vi "sub_hw-set.vi"(7 "cmd":T1=enum."AO 0v", 8 "error in":errorcluster, 10 "DUT Ch":i32, 11 "onoff":bool) -> (0 "error out":errorcluster)   [LabVIEW 2019]
uses:
  hw-control.ctl
  cmd_timer.ctl
  _ctrl/rw.ctl
  Devices/NI Board/cDAQ-9269 AO/type_signal.ctl
  Durability/common/UI.ctl
  Devices/NI Board/cDAQ-9476 DO/cnt_Relay.ctl
  Devices/NI Board/cDAQ-9476 DO/cnt_do.ctl
  Durability/common/cmd_timecheck.ctl
  _ctrl/BP4610_config.ctl
  _ctrl/BP4610_cmd.ctl
  _ctrl/DSP_action.ctl
  _ctrl/create-rw-close.ctl
  _ctrl/start.ctl
  _ctrl/fgv_DL950.ctl
  cmd_offtimecheck.ctl
  _ctrl/system-status.ctl
  _ctrl/init-r-stop.ctl
  4ec001e4-0f3b-4ebf-849a-f4f83a7bab7c.vi
  e6889d7c-de11-414d-a0e0-4227c0c1917b.vi
  0bae8188-c8c3-4ffc-ad07-b2da4a811416.vi
  23ae199e-3a96-4767-bc63-b89c967d0f14.vi
  470acc9e-1f4f-4ee6-a90f-225dc51f797d.vi
  0dce9dd1-3bd9-4495-8249-675a9cbc74d0.vi
  06f06628-476d-4804-93c1-d30ef29838a9.vi
  9f7e44c7-c157-4d85-83aa-43634e971710.vi
  Glob_Ref.vi
  Durability/common/Global 1.vi
  34f4878d-8da2-4261-96f6-505d6876a221.vi
  e9941be1-5017-49c9-9991-91539d334db2.vi
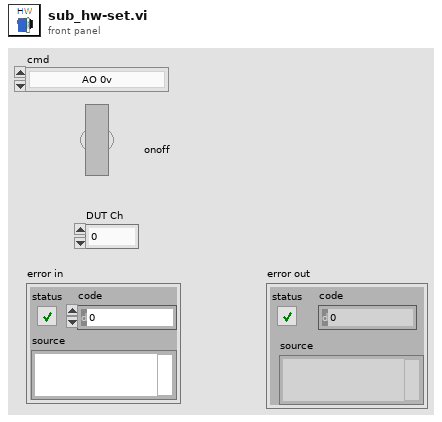
[diagram p1: front panel]
types:
  T1 = typedef "hw-control.ctl" = enum16{"DL950 ready", "DL950 clear", "DL950 trigger", "DL950 read", "DL950 read seq", "DL950 Tsingle query", "AO 12v", "AO wave", "AO 0v", "relay all-off", "Discharge check", "Discharge", "Relay1", "Relay2", "Relay3", "Relay4", "Relay5", "Relay6", "BP4610 onoff", "BP4610 set", "DSP1500 set", "DSP1500 onoff"}
  T2 = typedef "rw.ctl" = enum16{"read", "write"}
  T3 = typedef "cmd_timer.ctl" = enum16{"init", "init_update", "run", "default", "update"}
  T4 = typedef "cap_config.ctl" = cluster{"Test Mode":enum32{"6.3.2 저온 작동/방치 시험", "6.3.3 고온 작동/방치 시험", "6.3.4 온도 싸이클 시험", "6.3.6 온습도 싸이클 시험", "6.3.8 결로 시험", "6.3.9 빙결 시험"}, "ON time[ms]":dbl, "OFF time[ms]":dbl, "1. 작동시간[분]":dbl, "2. 미작동시간[분]":dbl, "3. 작동시간[분]":dbl, "level[V]":dbl, "duty":dbl, "Freq":dbl, "Voltage+[V]":dbl, "Voltage-[V]":dbl, "Current+[A]":dbl, "Current-[A]":dbl, "출력전압[V]":dbl, "출력전류[A]":dbl, "OVP Level":dbl, "OCP Level":dbl, "Time Div":u16, "Record Len":i32, "방전 기준[V]":dbl, "Repeate (Each Ch)":u32, "Cycle[N]":u32, "ON/OFF 회 수[N]":dbl, "TrigPos[%]":dbl, "시험시간[분]":dbl}
  T5 = typedef "Testing-info.ctl" = cluster{"전체채널수":u8, "현재채널번호":u8, "Irms":dbl, "입력전압":dbl, "입력전류":dbl, "출력전압":dbl, "출력전류":dbl, "온도":dbl, "제어단 단선":bool, "제어단 단락":bool, "제어단 특성변화":bool, "출력단 단선":bool, "출력단 단락":bool, "출력단 특성변화":bool, "출력단 전압":bool, "카운트 일치":bool, "Irms 판정":bool, "온도":bool, "테스트 회수":u32, "TestType":T6, "현재회수":u32, "Ch selection":cluster{"1ch":bool, "2ch":bool, "3ch":bool, "4ch":bool, "5ch":bool, "6ch":bool}, "반복":u32, "Path":path, "파일생성주기":u32, "start time":dbl, "stop time":dbl, "현재반복회수":u32, "NG":cluster{"입출력 카운트":bool, "출력전류RMS":bool}}
  T6 = typedef "sequence_single.ctl" = enum16{"Register", "RC", "B1", "B2", "B3", "Oper_LV", "Oper_HV", "ContR_LV"}
  T7 = typedef "type_signal.ctl" = enum16{"wave", "level"}
  T8 = typedef "UI.ctl" = enum16{"Alarm yellow", "DL950 graph show", "DL950 graph clear", "AO value", "AO blink onoff", "Discharge relay", "Input Power", "Outpower", "Relay in1", "Relay in2", "Relay in3", "Relay in4", "Relay in5", "Relay in6", "Relay out1", "Relay out2", "Relay out3", "Relay out4", "Relay out5", "Relay out6", "Relay all off"}
  T9 = typedef "cmd_timecheck.ctl" = enum16{"Group start", "Group end", "Grout dt", "Ch start", "Ch end", "Ch dt", "init", "NF start", "NF stop", "idrc start", "idrc stop", "scope start", "scope stop", "ao start", "ao stop", "relay start", "relay stop", "NF read start", "NF read stop", "NF set start", "NF set stop", "idrc level start", "idrc level stop", "scope trig start", "scope trig stop", "relay dischar star", "relay dischar stop", "data process start", "data process stop", "ch-relay on start", "ch-relay on stop", "hw set start", "hw set stop", "pwr-in on start", "pwr-in on stop", "pwr-out on start", "pwr-out on stop", "ao on start", "ao on stop", "ao 0v start", "ao 0v stop", "pwr-in off start", "pwr-in off stop", "relay-all off start", "relay-all off stop", "pwr-out off start", "pwr-out off stop", "discharge start", "discharge stop", "950 read start", "950 read stop"}
  T10 = typedef "cnt_do.ctl" = enum16{"open", "initial", "update", "run", "close"}
  T11 = typedef "cnt_Relay.ctl" = enum32{"R_Load", "R_out1", "R_out2", "R_out3", "R_out4", "R_out5", "R_out6", "R8", "R9", "R10", "R11", "R12", "R13", "R14", "R15", "R16", "R_in1", "R_in2", "R_in3", "R_in4", "R_in5", "R_in6", "R23", "R24", "R25", "R26", "R27", "R_red", "R_yellow", "R_green", "R_buz", "R_purple"}
  T12 = typedef "BP4610_cmd.ctl" = enum16{"open", "read", "set", "set_seq", "limit", "limit_seq", "output on", "output off", "close"}
  T13 = typedef "BP4610_config.ctl" = cluster{"VISA":refnum<visa-resource-name>, "Limit-BP":cluster{"Set":enum16{"Current", "Voltage"}, "Voltage+[V]":dbl, "Current+[A]":dbl, "Voltage-[V]":dbl, "Current-[A]":dbl}, "SET BP":cluster{"Set":enum16{"Current", "Voltage", "FREQ/WAVE"}, "Operation mode":u16, "Voltage[Vp-p]":dbl, "Current[Ap-p]":dbl, "Voltage[V]":dbl, "Current[A]":dbl, "Frequency[Hz]":dbl, "Waveform":enum16{"Sine", "Square", "ARB 1", "ARB 2", "ARB 3", "ARB 4", "ARB 5", "ARB 6", "ARB 7", "ARB 8", "ARB 9", "ARB 10", "ARB 11", "ARB 12", "ARB 13", "ARB 14", "ARB 15", "ARB 16"}}}
  T14 = typedef "DSP_action.ctl" = enum16{"False", "cont", "on", "off", "discont", "protection", "protection_seq", "preread", "level_seq", "level_m", "read", "stop", "exit"}
  T15 = typedef "start.ctl" = enum16{"init", "open", "set", "start", "stop", "read", "read_items", "query", "close", "T_single", "reset", "exit"}
  T16 = typedef "create-rw-close.ctl" = enum16{"create", "write", "read", "delete", "close"}
  T17 = typedef "fgv_DL950.ctl" = enum16{"init", "config", "Set-NCh", "setapply", "trigger", "history_clear", "read", "time-div", "wave-aquis", "start", "query", "abort", "set_items", "reset_items", "read_items", "percent_rise", "trigger_single", "stop", "offset cancel", "close"}
  T18 = typedef "cmd_offtimecheck.ctl" = enum16{"start", "check", "init"}
  T19 = typedef "system-status.ctl" = enum16{"Initial", "Update", "Clear", "Read"}
  T20 = typedef "init-r-stop.ctl" = enum16{"ini", "read", "stop"}
  T21 = typedef "Set_AO_Wave-config.ctl" = cluster{"offset":dbl, "Samples":i32, "duty":dbl, "Rate":dbl, "wfm":cluster{"Freq":dbl, "Amp":dbl, "Type":enum16{"Sine Wave", "Triangle Wave", "Square Wave", "Sawtooth Wave"}}}
  T22 = typedef "ref_all.ctl" = cluster{"BP4610 Config":refnum<vi>, "DSP1950 Config":refnum<vi>, "2470-config":refnum<vi>, "cDAQ 9269 AO config":refnum<vi>, "cDAQ 9221 Config":refnum<vi>, "cDAQ-9467 Config":refnum<vi>, "Waveform":refnum<vi>, "DL950 wfm":refnum<vi>, "AI Graph":refnum<vi>, "AO_Wave-config":refnum<vi>, "DL950 items":refnum<vi>, "Volt":refnum<vi>, "Current":refnum<vi>, "AO_Level":refnum<vi>, "RC-Test Judgement ":refnum<vi>, "Log path":refnum<vi>, "시험명":refnum<vi>, "file renew[Hr]":refnum<vi>, "Breakdown-Spec":refnum<vi>, "paste":refnum<vi>, "copy":refnum<vi>, "DL950_config":refnum<vi>, "종료시간":refnum<vi>, "경과시간":refnum<vi>, "Apply":refnum<vi>, "DSP Config LV ":refnum<vi>, "Testconfig":refnum<vi>}
  T23 = cluster{"Freq":dbl, "level[V]":dbl, "duty":dbl, "On time[ms]":dbl}
  T24 = typedef "cDAQ-9269 Config.ctl" = cluster{"Ch":tag, "Max V":dbl, "Min V":dbl, " Rate":dbl, "N pts":i32, "sample mode":i32}
  T25 = typedef "DSP_config.ctl" = cluster{"Port":refnum<visa-resource-name>, "OVP Level":dbl, "OCP Level":dbl, "Current":dbl, "Voltage":dbl}
  T26 = typedef "DL950_wfms.ctl" = cluster{"wfms":waveform(dbl)[], "Waveform_2":cluster{"t0":dbl, "dt":dbl, "Y":dbl[][]}, "items":dbl[][], "da950_array":dbl[]}
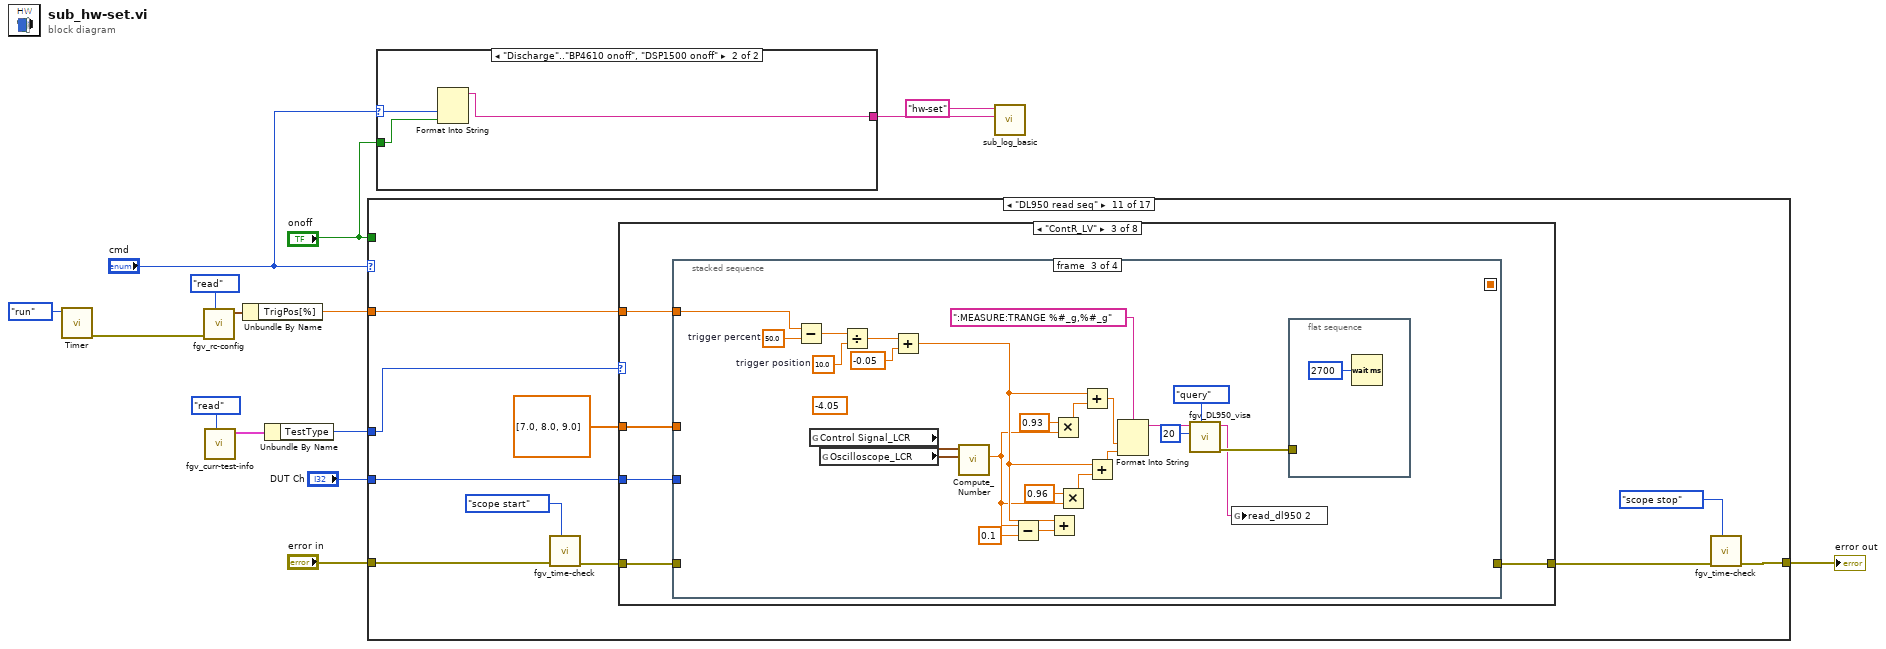
[diagram p0: block diagram]
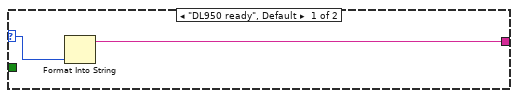
[diagram p2: hidden frame]
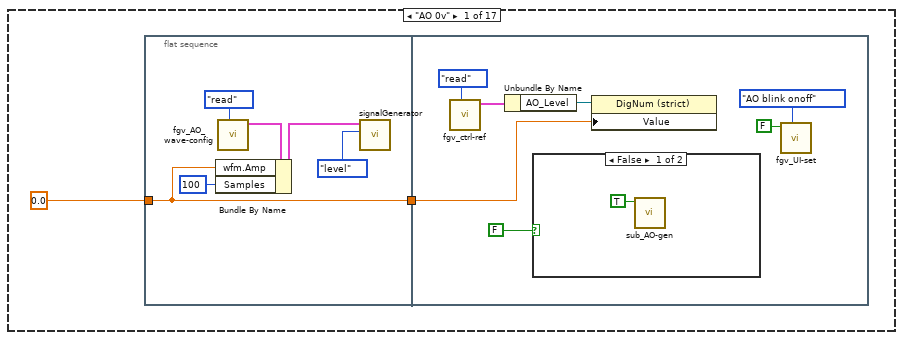
[diagram p3: hidden frame]
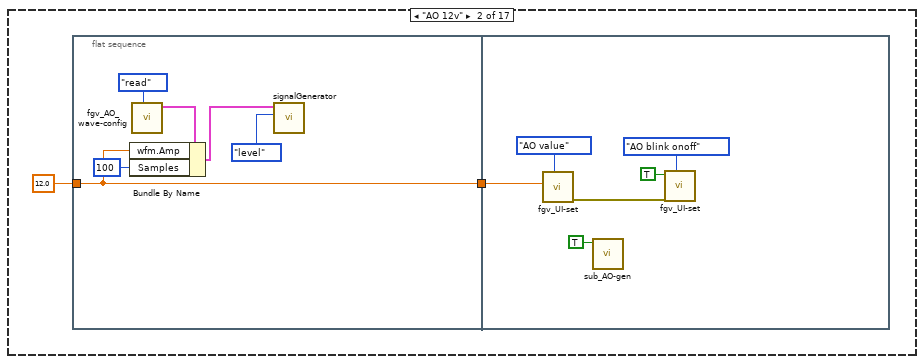
[diagram p5: hidden frame]
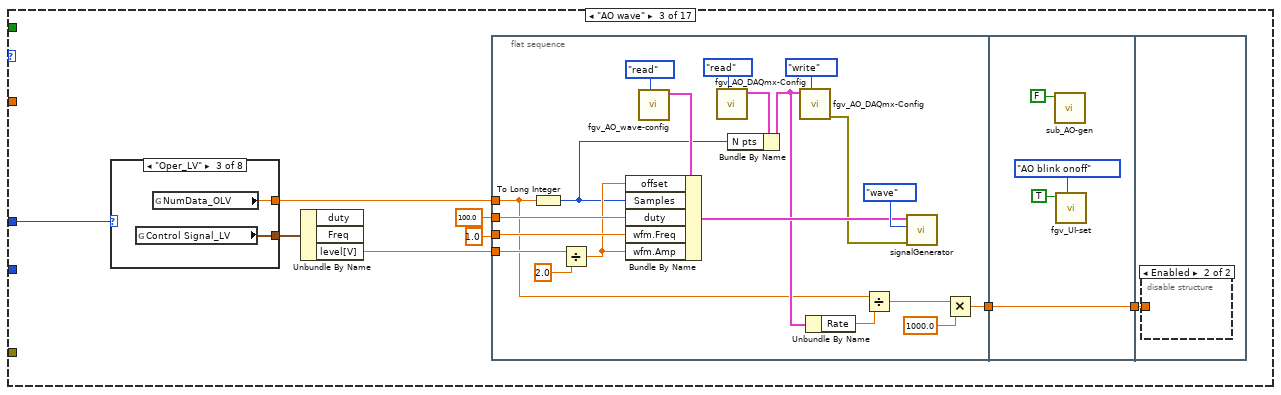
[diagram p6: hidden frame]
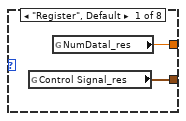
[diagram p7: hidden frame]
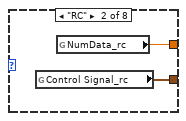
[diagram p8: hidden frame]
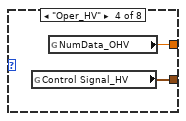
[diagram p9: hidden frame]
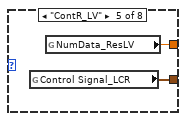
[diagram p10: hidden frame]
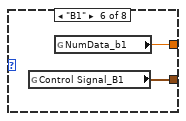
[diagram p11: hidden frame]
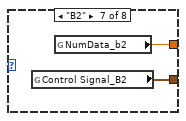
[diagram p12: hidden frame]
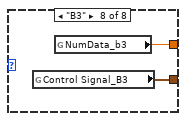
[diagram p13: hidden frame]
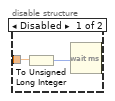
[diagram p14: hidden frame]
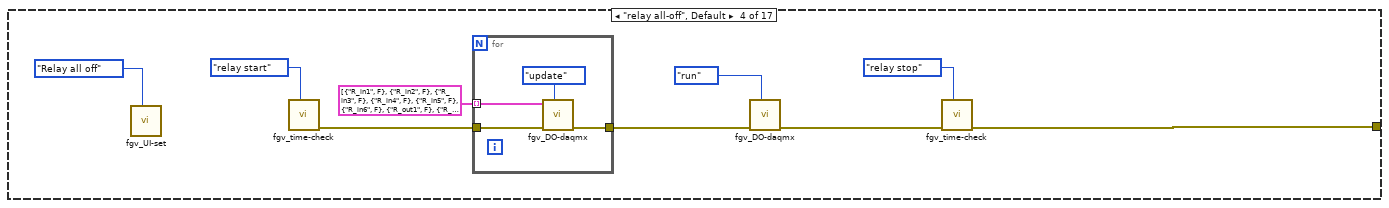
[diagram p15: hidden frame]
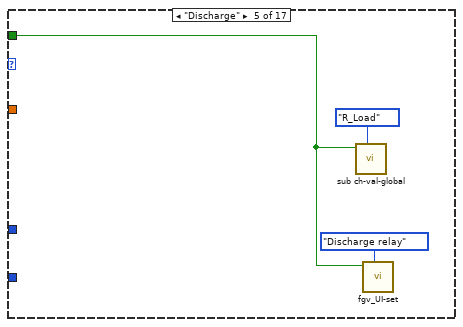
[diagram p16: hidden frame]
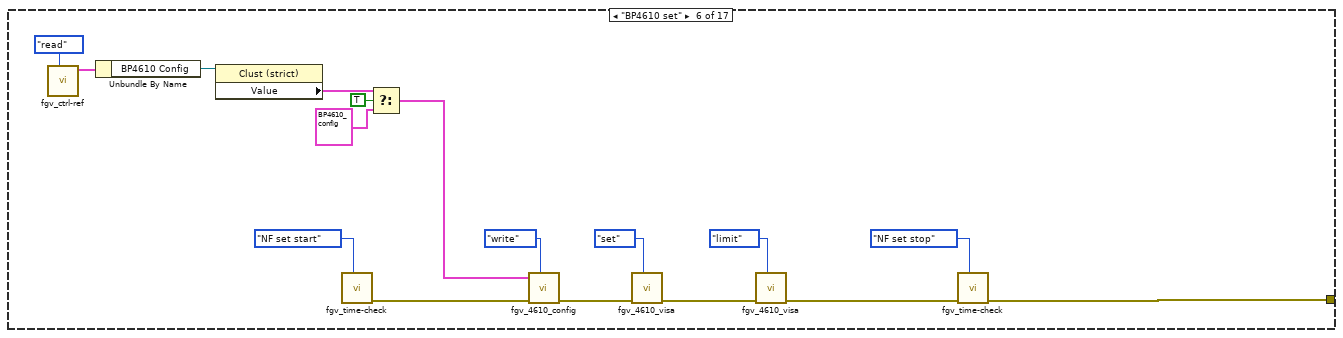
[diagram p17: hidden frame]
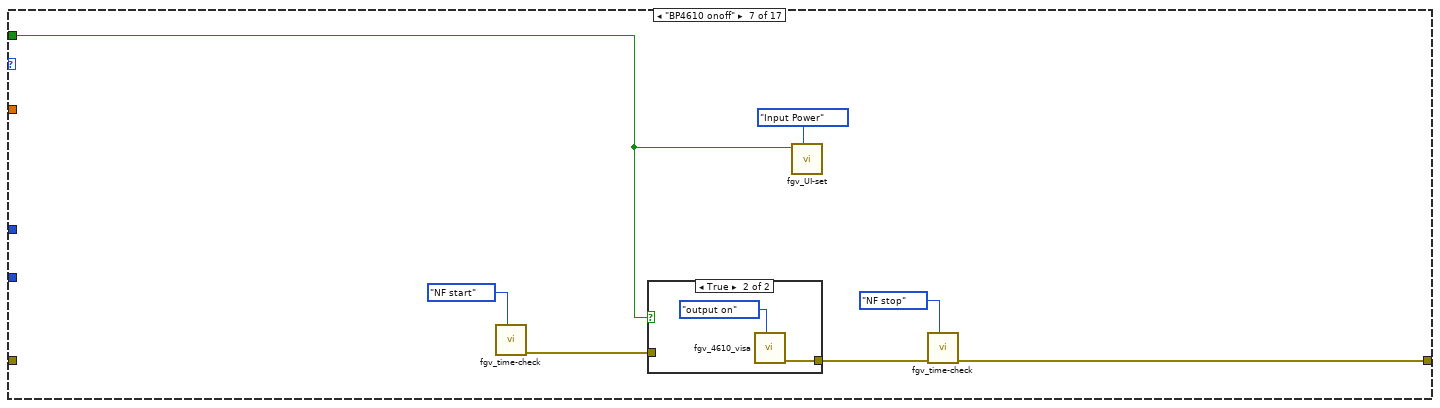
[diagram p18: hidden frame]
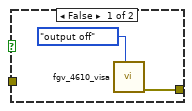
[diagram p19: hidden frame]
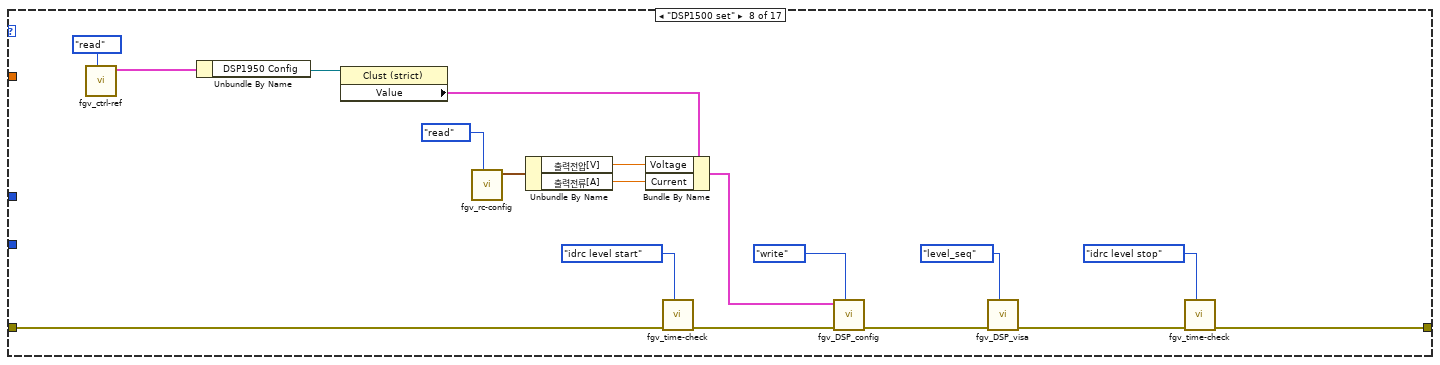
[diagram p20: hidden frame]
diagram:
  n1 = call "Timer.vi"("cmd"=cmd_timer."run") -> ("error out"=w2:errorcluster)  [unwired: 8 in, 2 out]
  n2 = call "fgv_rc-config.vi"("cmd"=rw."read", "error in (no error)"=w2) -> ("Testconfig out"=w5:T4)  [unwired: 8 in, 1 out]
  n3 = call "fgv_curr-test-info.vi"("cmd"=rw."read") -> ("현재테스트 정보 2"=w10:T5)  [unwired: 10 in]
  n4 = Unbundle By Name(w5) -> ("TrigPos[%]"=w3:dbl)
  n5 = Unbundle By Name(w10) -> ("TestType"=w9:T6)
  n6 = case shown="\"DL950 read seq\"" "cmd" {
    selector: "cmd" -> [_ _ _ _ _ _ _ _ _ _ _ _ _ _ w577 _ _]
    tunnel: "onoff" -> [_ _ _ _ w112 _ w136 _ w165 _ _ _ _ _ w581 _ _]
    tunnel: "DUT Ch" -> [_ _ _ _ _ _ _ _ _ _ w183 _ _ _ _ _ _]
    tunnel: w9 -> [_ _ w48 _ _ _ _ _ _ _ w175 _ _ _ _ _ w651]
    tunnel: "error in" -> [_ _ _ _ _ _ _ w141 _ _ w178 _ _ _ _ _ _]
    tunnel: [_ _ _ w97 _ w113 w130 w142 w159 _ w177 _ w536 w545 _ _ _] -> w7
    tunnel: w3 -> [_ _ _ _ _ _ _ _ _ _ w174 _ _ _ _ _ _]
    frame "AO 0v" {
      n7 = flat-sequence {
        tunnel: [w19] -> w17
        tunnel: 0.0 ("wfm.Amp") -> [w19]
        tunnel: w17 -> [w27]
        frame #0 {
          n8 = call "fgv_AO_wave-config.vi"("cmd"=rw."read") -> ("Square Wave 2"=w21:T21)  [unwired: 9 in, 1 out]
          n9 = Bundle By Name(cluster=w21, "wfm.Amp"=w19, "Samples"=100) -> (w20:T21)
          n10 = call "signalGenerator.vi"("cnt"=type_signal."level", "Square Wave"=w20) -> ()  [unwired: 8 in, 2 out]
        }
        frame #1 {
          n11 = call "fgv_ctrl-ref.vi"("cmd"=rw."read") -> ("output cluster 2"=w29:T22)  [unwired: 9 in, 1 out]
          n12 = Unbundle By Name(w29) -> ("AO_Level"=w28:refnum<vi>)
          n13 = case shown="False" FALSE {
            frame False {
              n14 = call "sub_AO-gen.vi"("level"=TRUE) -> ()  [unwired: 10 in, 1 out]
            }
            frame True {
            }
          }
          n15 = property class="DigNum (strict)"(reference=w28, "Value"=w27) -> ()  [unwired: 1 in, 2 out]
          n16 = call "fgv_UI-set.vi"("cmd"=UI."AO blink onoff", "onoff"=FALSE) -> ()  [unwired: 9 in, 1 out]
        }
      }
    }
    frame "AO 12v" {
      n17 = flat-sequence {
        tunnel: [w35] -> w33
        tunnel: 12.0 ("wfm.Amp") -> [w35]
        tunnel: w33 -> [w44]
        frame #0 {
          n18 = call "fgv_AO_wave-config.vi"("cmd"=rw."read") -> ("Square Wave 2"=w37:T21)  [unwired: 9 in, 1 out]
          n19 = Bundle By Name(cluster=w37, "wfm.Amp"=w35, "Samples"=100) -> (w36:T21)
          n20 = call "signalGenerator.vi"("cnt"=type_signal."level", "Square Wave"=w36) -> ()  [unwired: 8 in, 2 out]
        }
        frame #1 {
          n21 = call "fgv_UI-set.vi"("cmd"=UI."AO value", "Value"=w44) -> ("error out"=w41:errorcluster)  [unwired: 9 in]
          n22 = call "sub_AO-gen.vi"("level"=TRUE) -> ()  [unwired: 10 in, 1 out]
          n23 = call "fgv_UI-set.vi"("cmd"=UI."AO blink onoff", "error in"=w41, "onoff"=TRUE) -> ()  [unwired: 8 in, 1 out]
        }
      }
    }
    frame "AO wave" {
      n24 = case shown="\"Oper_LV\"" w48 {
        tunnel: [w55 w57 w59 w61 w63 w65 w67 w69] -> w53
        tunnel: [w54 w56 w58 w60 w62 w64 w66 w68] -> w51
        frame "Register", Default {
          n25 = global read "Glob_Ref.vi" "Control Signal_res"() -> (w55:T23)
          n26 = global read "Glob_Ref.vi" "NumDatal_res"() -> (w54:dbl)
        }
        frame "RC" {
          n27 = global read "Glob_Ref.vi" "Control Signal_rc"() -> (w57:T23)
          n28 = global read "Glob_Ref.vi" "NumData_rc"() -> (w56:dbl)
        }
        frame "Oper_LV" {
          n29 = global read "Glob_Ref.vi" "Control Signal_LV"() -> (w59:T23)
          n30 = global read "Glob_Ref.vi" "NumData_OLV"() -> (w58:dbl)
        }
        frame "Oper_HV" {
          n31 = global read "Glob_Ref.vi" "Control Signal_HV"() -> (w61:T23)
          n32 = global read "Glob_Ref.vi" "NumData_OHV"() -> (w60:dbl)
        }
        frame "ContR_LV" {
          n33 = global read "Glob_Ref.vi" "Control Signal_LCR"() -> (w63:T23)
          n34 = global read "Glob_Ref.vi" "NumData_ResLV"() -> (w62:dbl)
        }
        frame "B1" {
          n35 = global read "Glob_Ref.vi" "Control Signal_B1"() -> (w65:T23)
          n36 = global read "Glob_Ref.vi" "NumData_b1"() -> (w64:dbl)
        }
        frame "B2" {
          n37 = global read "Glob_Ref.vi" "Control Signal_B2"() -> (w67:T23)
          n38 = global read "Glob_Ref.vi" "NumData_b2"() -> (w66:dbl)
        }
        frame "B3" {
          n39 = global read "Glob_Ref.vi" "Control Signal_B3"() -> (w69:T23)
          n40 = global read "Glob_Ref.vi" "NumData_b3"() -> (w68:dbl)
        }
      }
      n41 = Unbundle By Name(w53) -> ("level[V]"=w52:dbl)  [unwired: 2 out]
      n42 = flat-sequence {
        tunnel: 100.0 ("duty") -> [w86]
        tunnel: 1.0 ("Freq") -> [w85]
        tunnel: w52 -> [w84]
        tunnel: w51 -> [w71]
        tunnel: [w72] -> w50
        tunnel: w50 -> [w91]
        tunnel: [w91] -> w49
        tunnel: w49 -> [w94]
        frame #0 {
          n43 = To Long Integer(number=w71) -> (32bit integer=w70:i32)
          n44 = Divide(x=w84, y=2.0) -> (x/y=w81:dbl)
          n45 = call "fgv_AO_wave-config.vi"("cmd"=rw."read") -> ("Square Wave 2"=w87:T21)  [unwired: 9 in, 1 out]
          n46 = Bundle By Name(cluster=w87, "offset"=w81, "Samples"=w70, "duty"=w86, "wfm.Freq"=w85, "wfm.Amp"=w81) -> (w82:T21)
          n47 = call "fgv_AO_DAQmx-Config.vi"("cmd"=rw."read") -> ("config 2"=w80:T24)  [unwired: 9 in, 1 out]
          n48 = Bundle By Name(cluster=w80, "N pts"=w70) -> (w76:T24)
          n49 = call "fgv_AO_DAQmx-Config.vi"("cmd"=rw."write", "9269 AO Config"=w76) -> ("error out"=w77:errorcluster)  [unwired: 8 in, 1 out]
          n50 = Unbundle By Name(w76) -> ("Rate"=w75:dbl)
          n51 = Divide(x=w71, y=w75) -> (x/y=w74:dbl)
          n52 = call "signalGenerator.vi"("error in"=w77, "cnt"=type_signal."wave", "Square Wave"=w82) -> ()  [unwired: 7 in, 2 out]
          n53 = Multiply(x=w74, y=1000.0) -> (x*y=w72:dbl)
        }
        frame #1 {
          n54 = call "sub_AO-gen.vi"("level"=FALSE) -> ()  [unwired: 10 in, 1 out]
          n55 = call "fgv_UI-set.vi"("cmd"=UI."AO blink onoff", "onoff"=TRUE) -> ()  [unwired: 9 in, 1 out]
        }
        frame #2 {
          n56 = disable-structure shown="Enabled" {
            disable-tunnel: w94 -> [w96 _]
            frame Disabled {
              n57 = To Unsigned Long Integer(number=w96) -> (unsigned 32bit integer=w95:u32)
              n58 = Wait (ms)(milliseconds to wait=w95) -> ()  [unwired: 1 out]
            }
            frame Enabled {
            }
          }
        }
      }
    }
    frame "relay all-off", Default {
      n59 = call "fgv_UI-set.vi"("cmd"=UI."Relay all off") -> ()  [unwired: 10 in, 1 out]
      n60 = call "fgv_time-check.vi"("cmd"=cmd_timecheck."relay start") -> ("error out"=w100:errorcluster)  [unwired: 9 in, 1 out]
      n61 = for {
        tunnel: cluster{"Relay":T11, "Boolean":bool}[] [{"Relay"=enum."R_in1", "Boolean"=FALSE}, {"Relay"=enum."R_in2", "Boolean"=FALSE}, {"Relay"=enum."R_in3", "Boolean"=FALSE}, {"Relay"=enum."R_in4", "Boolean"=FALSE}, {"Relay"=enum."R_in5", "Boolean"=FALSE}, {"Relay"=enum."R_in6", "Boolean"=FALSE}, {"Relay"=enum."R_out1", "Boolean"=FALSE}, {"Relay"=enum."R_out2", "Boolean"=FALSE}, {"Relay"=enum."R_out3", "Boolean"=FALSE}, {"Relay"=enum."R_out4", "Boolean"=FALSE}, {"Relay"=enum."R_out5", "Boolean"=FALSE}, {"Relay"=enum."R_out6", "Boolean"=FALSE}] -> [w109] mode=indexing
        tunnel: [w107] -> w102
        tunnel: w100 -> [w106]
        n62 = call "fgv_DO-daqmx.vi"("cnt"=cnt_do."update", "error in"=w106, "Relay"=w109) -> ("error out"=w107:errorcluster)  [unwired: 8 in]
      }
      n63 = call "fgv_DO-daqmx.vi"("cnt"=cnt_do."run", "error in"=w102) -> ("error out"=w98:errorcluster)  [unwired: 9 in]
      n64 = call "fgv_time-check.vi"("cmd"=cmd_timecheck."relay stop", "error in (no error)"=w98) -> ("error out"=w97:errorcluster)  [unwired: 8 in, 1 out]
    }
    frame "Discharge" {
      n65 = call "sub ch-val-global.vi"("Relay"=cnt_Relay."R_Load", "onoff"=w112) -> ()  [unwired: 10 in]
      n66 = call "fgv_UI-set.vi"("cmd"=UI."Discharge relay", "onoff"=w112) -> ()  [unwired: 9 in, 1 out]
    }
    frame "BP4610 set" {
      n67 = call "fgv_ctrl-ref.vi"("cmd"=rw."read") -> ("output cluster 2"=w127:T22)  [unwired: 9 in, 1 out]
      n68 = Unbundle By Name(w127) -> ("BP4610 Config"=w126:refnum<vi>)
      n69 = property class="Clust (strict)"(reference=w126) -> ("Value"=w125:T13)  [unwired: 1 in, 2 out]
      n70 = call "fgv_time-check.vi"("cmd"=cmd_timecheck."NF set start") -> ("error out"=w116:errorcluster)  [unwired: 9 in, 1 out]
      n71 = Select(t=w125, s=TRUE, f=T13 {"VISA"="USB0::0x0D4A::0x0040::9426270::INSTR", "Limit-BP"={"Set"=enum."Current", "Voltage+[V]"=20.0, "Current+[A]"=5.0, "Voltage-[V]"=-20.0, "Current-[A]"=-5.0}, "SET BP"={"Set"=enum."Voltage", "Operation mode"=1, "Voltage[Vp-p]"=20.0, "Current[Ap-p]"=5.0, "Voltage[V]"=12.0, "Current[A]"=5.0, "Frequency[Hz]"=100.0, "Waveform"=enum."Square"}} ("BP4610 Config 2")) -> (s? t:f=w122:T13)
      n72 = call "fgv_4610_config.vi"("cmd"=rw."write", "error in (no error)"=w116, "BP4610 Config"=w122) -> ("error out"=w119:errorcluster)  [unwired: 7 in, 1 out]
      n73 = call "fgv_4610_visa.vi"("cmd"=BP4610_cmd."set", "error in"=w119) -> ("error out"=w118:errorcluster)  [unwired: 9 in]
      n74 = call "fgv_4610_visa.vi"("cmd"=BP4610_cmd."limit", "error in"=w118) -> ("error out"=w114:errorcluster)  [unwired: 9 in]
      n75 = call "fgv_time-check.vi"("cmd"=cmd_timecheck."NF set stop", "error in (no error)"=w114) -> ("error out"=w113:errorcluster)  [unwired: 8 in, 1 out]
    }
    frame "BP4610 onoff" {
      n76 = call "fgv_time-check.vi"("cmd"=cmd_timecheck."NF start") -> ("error out"=w134:errorcluster)  [unwired: 9 in, 1 out]
      n77 = case shown="True" w136 {
        tunnel: w134 -> [_ _]
        tunnel: [w137 w139] -> w132
        frame False {
          n78 = call "fgv_4610_visa.vi"("cmd"=BP4610_cmd."output off") -> ("error out"=w137:errorcluster)  [unwired: 10 in]
        }
        frame True {
          n79 = call "fgv_4610_visa.vi"("cmd"=BP4610_cmd."output on") -> ("error out"=w139:errorcluster)  [unwired: 10 in]
        }
      }
      n80 = call "fgv_UI-set.vi"("cmd"=UI."Input Power", "onoff"=w136) -> ()  [unwired: 9 in, 1 out]
      n81 = call "fgv_time-check.vi"("cmd"=cmd_timecheck."NF stop", "error in (no error)"=w132) -> ("error out"=w130:errorcluster)  [unwired: 8 in, 1 out]
    }
    frame "DSP1500 set" {
      n82 = call "fgv_ctrl-ref.vi"("cmd"=rw."read") -> ("output cluster 2"=w155:T22)  [unwired: 9 in, 1 out]
      n83 = Unbundle By Name(w155) -> ("DSP1950 Config"=w154:refnum<vi>)
      n84 = property class="Clust (strict)"(reference=w154) -> ("Value"=w151:T25)  [unwired: 1 in, 2 out]
      n85 = call "fgv_rc-config.vi"("cmd"=rw."read") -> ("Testconfig out"=w152:T4)  [unwired: 9 in, 1 out]
      n86 = Unbundle By Name(w152) -> ("출력전압[V]"=w150:dbl, "출력전류[A]"=w149:dbl)
      n87 = Bundle By Name(cluster=w151, "Voltage"=w150, "Current"=w149) -> (w148:T25)
      n88 = call "fgv_time-check.vi"("cmd"=cmd_timecheck."idrc level start", "error in (no error)"=w141) -> ("error out"=w146:errorcluster)  [unwired: 8 in, 1 out]
      n89 = call "fgv_DSP_config.vi"("cmd"=rw."write", "error in (no error)"=w146, "DSP Config HV IN"=w148) -> ("error out"=w157:errorcluster)  [unwired: 6 in, 2 out]
      n90 = call "fgv_DSP_visa.vi"("action"=DSP_action."level_seq", "error in"=w157) -> ("error out"=w144:errorcluster)  [unwired: 9 in]
      n91 = call "fgv_time-check.vi"("cmd"=cmd_timecheck."idrc level stop", "error in (no error)"=w144) -> ("error out"=w142:errorcluster)  [unwired: 8 in, 1 out]
    }
    frame "DSP1500 onoff" {
      n92 = call "fgv_time-check.vi"("cmd"=cmd_timecheck."idrc start") -> ("error out"=w163:errorcluster)  [unwired: 9 in, 1 out]
      n93 = case shown="False" w165 {
        tunnel: w163 -> [w167 w169]
        tunnel: [w166 w170] -> w162
        frame False {
          n94 = call "fgv_DSP_visa.vi"("action"=DSP_action."off", "error in"=w167) -> ("error out"=w166:errorcluster)  [unwired: 9 in]
        }
        frame True {
          n95 = call "fgv_DSP_visa.vi"("action"=DSP_action."on", "error in"=w169) -> ("error out"=w170:errorcluster)  [unwired: 9 in]
        }
      }
      n96 = call "fgv_UI-set.vi"("cmd"=UI."Outpower", "onoff"=w165) -> ()  [unwired: 9 in, 1 out]
      n97 = call "fgv_time-check.vi"("cmd"=cmd_timecheck."idrc stop", "error in (no error)"=w162) -> ("error out"=w159:errorcluster)  [unwired: 8 in, 1 out]
    }
    frame "DL950 read" {
      n98 = call "fgv_DL950_q.vi"("cmd"=create-rw-close."write", "data"=start."read") -> ()  [unwired: 8 in, 2 out]
    }
    frame "DL950 read seq" {
      n99 = call "fgv_time-check.vi"("cmd"=cmd_timecheck."scope start", "error in (no error)"=w178) -> ("error out"=w179:errorcluster)  [unwired: 8 in, 1 out]
      n100 = case shown="\"ContR_LV\"" w175 {
        tunnel: w183 -> [w190 w210 w242 w303 w364 w423 w486 w509]
        tunnel: [w184 w208 w239 w304 w365 w424 w480 w503] -> w180
        tunnel: w179 -> [w186 w209 w241 w304 w365 w424 w482 w505]
        tunnel: dbl[] [7.0, 8.0, 9.0] -> [_ w207 w240 w302 _ _ _ _]
        tunnel: w174 -> [_ _ w238 _ _ _ _ _]
        frame "Register", Default {
          # "46"
          n101 = call "Stall Data Flow.vim"("value in"=w186, "milliseconds to wait"=u32 2500) -> ("value out"=w185:errorcluster)  [unwired: 1 out]
          n102 = Index Array(array=dbl[] [9.0, 10.0, 11.0, 12.0, 13.0, 14.0], index=w190) -> (element=w193:dbl)
          n103 = Format Into String(format string=":MEASURE:CHANNEL5:PNUMber:VALUE?\n:MEASURE:CHANNEL6:PNUMber:VALUE?\n:MEASURE:CHANNEL4:RMS:VALUE?\n:MEASURE:CHANNEL5:RMS:VALUE?\n:MEASURE:CHANNEL6:RMS:VALUE?\n:MEASURE:CHANNEL%#_g:AVERage:VALUE?\n:MEASURE:CHANNEL6:LOW:VALUE?" ("String"), w193) -> (resulting string=w189:string)  [unwired: 2 in, 1 out]
          n104 = call "fgv_DL950_visa.vi"("cmd"=fgv_DL950."query", "error in"=w185, "ms"=u32 100, "Initiate"=w189) -> ("error out"=w194:errorcluster)  [unwired: 5 in, 2 out]
          n105 = call "Stall Data Flow.vim"("value in"=w194, "milliseconds to wait"=u32 100) -> ("value out"=w188:errorcluster)  [unwired: 1 out]
          n106 = call "TrangeCalc.vi"("error in (no error)"=w188) -> ("error out"=w184:errorcluster, "array"=w197:dbl[])  [unwired: 6 in, 2 out]
          n107 = call "fgv_950_parsing-arr.vi"("cmd"=rw."read") -> ("950 parsing arr 2"=w203:cluster{"950-arr 1":dbl[], "950-arr 2":dbl[]})  [unwired: 10 in]
          n108 = Bundle By Name(cluster=w203, "950-arr 1"=w197) -> (w202:cluster{"950-arr 1":dbl[], "950-arr 2":dbl[]})
          n109 = call "fgv_DL950_data.vi"("cmd"=rw."read") -> ("DL950 wfm 2"=w199:T26)  [unwired: 9 in, 1 out]
          n110 = Bundle By Name(cluster=w199, "da950_array"=w197) -> (w198:T26)
          n111 = call "fgv_950_parsing-arr.vi"("cmd"=rw."write", "950 parsing arr"=w202) -> ()  [unwired: 9 in, 1 out]
          n112 = call "fgv_DL950_data.vi"("cmd"=rw."write", "DL950 wfm"=w198) -> ()  [unwired: 8 in, 2 out]
        }
        frame "Oper_LV" {
          n113 = stacked-sequence {
            tunnel: w210 -> [_ w218]
            tunnel: w209 -> [_ w216]
            tunnel: [_ w214] -> w208
            tunnel: w207 -> [_ w213]
            frame #0 {
              n114 = call "Trig_TimeCheck.vi"("cmd"=cmd_offtimecheck."check") -> ()  [unwired: 10 in, 1 out]
            }
            frame #1 {
              n115 = disable-structure shown="Enabled" {
                disable-tunnel: w216 -> [w235 w237]
                disable-tunnel: [w234 w237] -> w215
                frame Disabled {
                  n116 = call "Stall Data Flow.vim"("value in"=w235, "milliseconds to wait"=u32 2500) -> ("value out"=w234:errorcluster)  [unwired: 1 out]
                }
                frame Enabled {
                }
              }
              n117 = Index Array(array=w213, index=w218) -> (element=w220:dbl)
              n118 = Format Into String(format string=":MEASURE:CHANNEL5:PNUMber:VALUE?\n:MEASURE:CHANNEL6:PNUMber:VALUE?\n:MEASURE:CHANNEL4:RMS:VALUE?\n:MEASURE:CHANNEL5:RMS:VALUE?\n:MEASURE:CHANNEL6:RMS:VALUE?\n:MEASURE:CHANNEL%#_g:AVERage:VALUE?\n:MEASURE:CHANNEL6:LOW:VALUE?" ("String"), w220) -> (resulting string=w217:string)  [unwired: 2 in, 1 out]
              n119 = call "fgv_DL950_visa.vi"("cmd"=fgv_DL950."query", "error in"=w215, "ms"=u32 50, "Initiate"=w217) -> ("error out"=w221:errorcluster)  [unwired: 5 in, 2 out]
              n120 = call "Stall Data Flow.vim"("value in"=w221, "milliseconds to wait"=u32 100) -> ("value out"=w212:errorcluster)  [unwired: 1 out]
              n121 = call "TrangeCalc.vi"("error in (no error)"=w212) -> ("error out"=w214:errorcluster, "array"=w224:dbl[])  [unwired: 6 in, 2 out]
              n122 = call "fgv_950_parsing-arr.vi"("cmd"=rw."read") -> ("950 parsing arr 2"=w230:cluster{"950-arr 1":dbl[], "950-arr 2":dbl[]})  [unwired: 10 in]
              n123 = Bundle By Name(cluster=w230, "950-arr 1"=w224) -> (w229:cluster{"950-arr 1":dbl[], "950-arr 2":dbl[]})
              n124 = call "fgv_DL950_data.vi"("cmd"=rw."read") -> ("DL950 wfm 2"=w226:T26)  [unwired: 9 in, 1 out]
              n125 = Bundle By Name(cluster=w226, "da950_array"=w224) -> (w225:T26)
              n126 = call "fgv_950_parsing-arr.vi"("cmd"=rw."write", "950 parsing arr"=w229) -> ()  [unwired: 9 in, 1 out]
              n127 = call "fgv_DL950_data.vi"("cmd"=rw."write", "DL950 wfm"=w225) -> ()  [unwired: 8 in, 2 out]
            }
          }
        }
        frame "ContR_LV" {
          n128 = stacked-sequence {
            seq-local: [_ w244 _ _] -> [_ _ _ w298]
            tunnel: w242 -> [_ w250 _ _]
            tunnel: w241 -> [_ w248 _ _]
            tunnel: w240 -> [_ w246 _ _]
            tunnel: [_ _ _ w287] -> w239
            tunnel: w238 -> [_ _ w267 _]
            frame #0 {
              n129 = call "Trig_TimeCheck.vi"("cmd"=cmd_offtimecheck."check") -> ()  [unwired: 10 in, 1 out]
            }
            frame #1 {
              n130 = disable-structure shown="Disabled" {
                disable-tunnel: w248 -> [w258 w260]
                disable-tunnel: [w257 w260] -> w247
                frame Disabled {
                  n131 = call "Stall Data Flow.vim"("value in"=w258, "milliseconds to wait"=u32 2500) -> ("value out"=w257:errorcluster)  [unwired: 1 out]
                }
                frame Enabled {
                }
              }
              n132 = Index Array(array=w246, index=w250) -> (element=w252:dbl)
              n133 = Format Into String(format string=":MEASURE:CHANNEL5:PNUMber:VALUE?\n:MEASURE:CHANNEL6:PNUMber:VALUE?\n:MEASURE:CHANNEL5:RMS:VALUE?\n:MEASURE:CHANNEL6:RMS:VALUE?\n:MEASURE:CHANNEL%#_g:AVERage:VALUE?" ("String"), w252) -> (resulting string=w249:string)  [unwired: 2 in, 1 out]
              n134 = call "fgv_DL950_visa.vi"("cmd"=fgv_DL950."query", "error in"=w247, "ms"=u32 50, "Initiate"=w249) -> ("error out"=w253:errorcluster)  [unwired: 5 in, 2 out]
              n135 = call "Stall Data Flow.vim"("value in"=w253, "milliseconds to wait"=u32 20) -> ("value out"=w245:errorcluster)  [unwired: 1 out]
              n136 = call "TrangeCalc.vi"("error in (no error)"=w245) -> ("array"=w244:dbl[])  [unwired: 6 in, 3 out]
            }
            frame #2 {
              w270 = 10.0  # trigger position
              w269 = 50.0  # trigger percent
              (unwired) -4.05 ("x")
              n137 = Subtract(x=w267, y=w269) -> (x-y=w266:dbl)
              n138 = global read "Glob_Ref.vi" "Control Signal_LCR"() -> (w282:T23)
              n139 = global read "Glob_Ref.vi" "Oscilloscope_LCR"() -> (w281:cluster{"Record Len":i32, "Time Div":u16})
              n140 = Divide(x=w266, y=w270) -> (x/y=w268:dbl)
              n141 = Add(x=w268, y=-0.05) -> (x+y=w263:dbl)
              n142 = call "Compute_Number.vi"("Oscilloscope"=w281, "Control Signal"=w282) -> ("NumDiv"=w261:dbl)  [unwired: 6 in, 3 out]
              n143 = Subtract(x=w261, y=0.1) -> (x-y=w274:dbl)
              n144 = Add(x=w263, y=w274) -> ()  [unwired: 1 out]
              n145 = Multiply(x=0.93, y=w261) -> (x*y=w283:dbl)
              n146 = Multiply(x=0.96, y=w261) -> (x*y=w265:dbl)
              n147 = Add(x=w263, y=w283) -> (x+y=w284:dbl)
              n148 = Add(x=w263, y=w265) -> (x+y=w262:dbl)
              n149 = Format Into String(format string=":MEASURE:TRANGE %#_g,%#_g" ("String"), w284, w262) -> (resulting string=w276:string)  [unwired: 2 in, 1 out]
              n150 = call "fgv_DL950_visa.vi"("cmd"=fgv_DL950."query", "ms"=u32 20, "Initiate"=w276) -> ("error out"=w273:errorcluster, "Data"=w272:string)  [unwired: 6 in, 1 out]
              n151 = global write "Global 1.vi" "read_dl950 2"(w272) -> ()
              n152 = flat-sequence {
                tunnel: w273 -> [_]
                frame #0 {
                  n153 = Wait (ms)(milliseconds to wait=u32 2700) -> ()  [unwired: 1 out]
                }
              }
            }
            frame #3 {
              n154 = call "fgv_DL950_visa.vi"("cmd"=fgv_DL950."query", "ms"=u32 20, "Initiate"=":MEASURE:CHANNEL3:AVERage:VALUE?\n:MEASURE:CHANNEL4:AVERage:VALUE?\n:MEASURE:CHANNEL6:AVERage:VALUE?" ("String")) -> ("error out"=w286:errorcluster)  [unwired: 6 in, 2 out]
              n155 = call "TrangeCalc.vi"("error in (no error)"=w286) -> ("error out"=w287:errorcluster, "array"=w297:dbl[])  [unwired: 6 in, 2 out]
              n156 = Build Array (concatenate)(w298, w297) -> (w288:dbl[])
              n157 = call "fgv_950_parsing-arr.vi"("cmd"=rw."read") -> ("950 parsing arr 2"=w296:cluster{"950-arr 1":dbl[], "950-arr 2":dbl[]})  [unwired: 10 in]
              n158 = Bundle By Name(cluster=w296, "950-arr 1"=w288) -> (w295:cluster{"950-arr 1":dbl[], "950-arr 2":dbl[]})
              n159 = call "fgv_DL950_data.vi"("cmd"=rw."read") -> ("DL950 wfm 2"=w294:T26)  [unwired: 9 in, 1 out]
              n160 = Bundle By Name(cluster=w294, "da950_array"=w288) -> (w293:T26)
              n161 = call "fgv_950_parsing-arr.vi"("cmd"=rw."write", "950 parsing arr"=w295) -> ()  [unwired: 9 in, 1 out]
              n162 = call "fgv_DL950_data.vi"("cmd"=rw."write", "DL950 wfm"=w293) -> ()  [unwired: 8 in, 2 out]
            }
          }
        }
        frame "Oper_HV" {
          n163 = stacked-sequence {
            seq-local: [w307 _ _ _ _ _ _] -> [_ w317 _ _ _ _ _]
            seq-local: [_ w315 _ _ _ _ _] -> [_ _ _ w333 _ _ _]
            tunnel: w303 -> [w308 _ _ _ w342 _ _]
            tunnel: w302 -> [w306 _ _ _ _ _ _]
            frame #0 {
              n164 = global read "Glob_Ref.vi" "NumDiv_rc"() -> (w310:dbl)
              n165 = disable-structure shown="Disabled" {
                frame Disabled {
                  n166 = Wait (ms)(milliseconds to wait=u32 500) -> ()  [unwired: 1 out]
                }
                frame Enabled {
                }
              }
              n167 = Index Array(array=w306, index=w308) -> (element=w311:dbl)
              n168 = Add(x=-4.05, y=w310) -> ()  [unwired: 1 out]
              n169 = call "Trig_TimeCheck.vi"("cmd"=cmd_offtimecheck."check") -> ()  [unwired: 10 in, 1 out]
              n170 = Format Into String(format string=":MEASURE:CHANNEL%#_g:AVERage:VALUE?", w311) -> (resulting string=w307:string)  [unwired: 2 in, 1 out]
            }
            frame #1 {
              n171 = Concatenate Strings(":TRIGGER:POSITION?\n:TIMebase:TDIV?\n:MEASURE:CHANNEL1:RISE:VALUE?\n:MEASURE:CHANNEL2:RISE:VALUE?\n:MEASURE:CHANNEL6:FALL:VALUE?\n:MEASURE:CHANNEL5:RMS:VALUE?\n:MEASURE:CHANNEL6:RMS:VALUE?\n:MEASURE:CHANNEL5:PNUMber:VALUE?" ("String"), "\n", w317) -> (w316:string)
              n172 = Wait (ms)(milliseconds to wait=u32 200) -> ()  [unwired: 1 out]
              n173 = call "fgv_DL950_visa.vi"("cmd"=fgv_DL950."query", "ms"=u32 20, "Initiate"=w316) -> ("error out"=w320:errorcluster, "Data"=w314:string)  [unwired: 6 in, 1 out]
              n174 = global write "Global 1.vi" "read_dl950 2"(w314) -> ()
              n175 = call "TrangeCalc.vi"("error in (no error)"=w320) -> ("T2"=w329:dbl, "T1"=w328:dbl, "array"=w315:dbl[])  [unwired: 6 in, 1 out]
              n176 = Format Into String(format string=":MEASURE:TRANGE %#_g,%#_g", w328, w329) -> (resulting string=w321:string)  [unwired: 2 in, 1 out]
              n177 = call "fgv_DL950_visa.vi"("cmd"=fgv_DL950."query", "ms"=u32 20, "Initiate"=w321) -> ()  [unwired: 6 in, 3 out]
            }
            frame #2 {
              n178 = Wait (ms)(milliseconds to wait=u32 2500) -> ()  [unwired: 1 out]
            }
            frame #3 {
              n179 = call "fgv_DL950_visa.vi"("cmd"=fgv_DL950."query", "ms"=u32 50, "Initiate"=":MEASURE:CHANNEL3:AVERage:VALUE?\n:MEASURE:CHANNEL4:AVERage:VALUE?\n:MEASURE:CHANNEL6:AVERage:VALUE?" ("format string")) -> ("error out"=w339:errorcluster)  [unwired: 6 in, 2 out]
              n180 = call "TrangeCalc.vi"("error in (no error)"=w339) -> ("array"=w332:dbl[])  [unwired: 6 in, 3 out]
              n181 = Build Array (concatenate)(w333, w332) -> (w331:dbl[])
              n182 = call "fgv_DL950_data.vi"("cmd"=rw."read") -> ("DL950 wfm 2"=w335:T26)  [unwired: 9 in, 1 out]
              n183 = Bundle By Name(cluster=w335, "da950_array"=w331) -> (w334:T26)
              n184 = call "fgv_DL950_data.vi"("cmd"=rw."write", "DL950 wfm"=w334) -> ()  [unwired: 8 in, 2 out]
            }
            frame #4 {
              n185 = disable-structure shown="Enabled" {
                disable-tunnel: w342 -> [w351 _]
                frame Disabled {
                  n186 = Index Array(array=dbl[] [9.0, 10.0, 11.0, 12.0, 13.0, 14.0], index=w351) -> (element=w346:dbl)
                  n187 = global read "Glob_Ref.vi" "NumDiv_rc"() -> (w345:dbl)
                  n188 = Add(x=-4.05, y=w345) -> (x+y=w343:dbl)
                  n189 = Format Into String(format string=":MEASURE:TRANGE -4.1,%#_g\n:MEASURE:CHANNEL%#_g:AVERage:VALUE?", w343, w346) -> (resulting string=w347:string)  [unwired: 2 in, 1 out]
                  n190 = call "fgv_DL950_visa.vi"("cmd"=fgv_DL950."query", "ms"=u32 110, "Initiate"=w347) -> ()  [unwired: 6 in, 3 out]
                }
                frame Enabled {
                }
              }
            }
            frame #5 {
              n191 = disable-structure shown="Disabled" {
                frame Disabled {
                  n192 = Wait (ms)(milliseconds to wait=u32 2000) -> ()  [unwired: 1 out]
                }
                frame Enabled {
                }
              }
            }
            frame #6 {
              n193 = disable-structure shown="Disabled" {
                frame Disabled {
                  n194 = call "fgv_950_parsing-arr.vi"("cmd"=rw."read") -> ("950 parsing arr 2"=w361:cluster{"950-arr 1":dbl[], "950-arr 2":dbl[]})  [unwired: 10 in]
                  n195 = Unbundle(w361) -> ("950-arr 1"=w362:dbl[], "950-arr 2"=w363:dbl[])
                  n196 = call "TrangeCalc.vi"() -> ("array"=w360:dbl[])  [unwired: 7 in, 3 out]
                  n197 = Build Array (concatenate)(w362, w363, w360) -> (w355:dbl[])
                  n198 = global write "Global 1.vi" "da950_array"(w355) -> ()
                  n199 = call "fgv_DL950_data.vi"("cmd"=rw."read") -> ("DL950 wfm 2"=w356:T26)  [unwired: 9 in, 1 out]
                  n200 = Bundle By Name(cluster=w356, "da950_array"=w355) -> (w354:T26)
                  n201 = call "fgv_DL950_data.vi"("cmd"=rw."write", "DL950 wfm"=w354) -> ()  [unwired: 8 in, 2 out]
                }
                frame Enabled {
                }
              }
            }
          }
        }
        frame "RC" {
          n202 = stacked-sequence {
            seq-local: [w366 _ _ _ _ _ _] -> [_ w376 _ _ _ _ _]
            seq-local: [_ w374 _ _ _ _ _] -> [_ _ _ w392 _ _ _]
            tunnel: w364 -> [w367 _ _ _ w401 _ _]
            frame #0 {
              n203 = global read "Glob_Ref.vi" "NumDiv_rc"() -> (w369:dbl)
              n204 = Index Array(array=dbl[] [9.0, 10.0, 11.0, 12.0, 13.0, 14.0], index=w367) -> (element=w370:dbl)
              n205 = Add(x=-4.05, y=w369) -> ()  [unwired: 1 out]
              n206 = Wait (ms)(milliseconds to wait=u32 500) -> ()  [unwired: 1 out]
              n207 = Format Into String(format string=":MEASURE:CHANNEL%#_g:AVERage:VALUE?", w370) -> (resulting string=w366:string)  [unwired: 2 in, 1 out]
            }
            frame #1 {
              n208 = Concatenate Strings(":TRIGGER:POSITION?\n:TIMebase:TDIV?\n:MEASURE:CHANNEL1:RISE:VALUE?\n:MEASURE:CHANNEL2:RISE:VALUE?\n:MEASURE:CHANNEL6:FALL:VALUE?\n:MEASURE:CHANNEL5:RMS:VALUE?\n:MEASURE:CHANNEL6:RMS:VALUE?\n:MEASURE:CHANNEL5:PNUMber:VALUE?" ("String"), "\n", w376) -> (w375:string)
              n209 = Wait (ms)(milliseconds to wait=u32 200) -> ()  [unwired: 1 out]
              n210 = call "fgv_DL950_visa.vi"("cmd"=fgv_DL950."query", "ms"=u32 20, "Initiate"=w375) -> ("error out"=w379:errorcluster)  [unwired: 6 in, 2 out]
              n211 = call "TrangeCalc.vi"("error in (no error)"=w379) -> ("T2"=w388:dbl, "T1"=w387:dbl, "array"=w374:dbl[])  [unwired: 6 in, 1 out]
              n212 = Format Into String(format string=":MEASURE:TRANGE %#_g,%#_g", w387, w388) -> (resulting string=w380:string)  [unwired: 2 in, 1 out]
              n213 = call "fgv_DL950_visa.vi"("cmd"=fgv_DL950."query", "ms"=u32 20, "Initiate"=w380) -> ()  [unwired: 6 in, 3 out]
            }
            frame #2 {
              n214 = Wait (ms)(milliseconds to wait=u32 2500) -> ()  [unwired: 1 out]
            }
            frame #3 {
              n215 = call "fgv_DL950_visa.vi"("cmd"=fgv_DL950."query", "ms"=u32 200, "Initiate"=":MEASURE:CHANNEL3:AVERage:VALUE?\n:MEASURE:CHANNEL4:AVERage:VALUE?\n:MEASURE:CHANNEL6:AVERage:VALUE?" ("format string")) -> ("error out"=w398:errorcluster)  [unwired: 6 in, 2 out]
              n216 = call "TrangeCalc.vi"("error in (no error)"=w398) -> ("array"=w391:dbl[])  [unwired: 6 in, 3 out]
              n217 = Build Array (concatenate)(w392, w391) -> (w390:dbl[])
              n218 = call "fgv_DL950_data.vi"("cmd"=rw."read") -> ("DL950 wfm 2"=w394:T26)  [unwired: 9 in, 1 out]
              n219 = Bundle By Name(cluster=w394, "da950_array"=w390) -> (w393:T26)
              n220 = call "fgv_DL950_data.vi"("cmd"=rw."write", "DL950 wfm"=w393) -> ()  [unwired: 8 in, 2 out]
            }
            frame #4 {
              n221 = disable-structure shown="Disabled" {
                disable-tunnel: w401 -> [w410 _]
                frame Disabled {
                  n222 = Index Array(array=dbl[] [9.0, 10.0, 11.0, 12.0, 13.0, 14.0], index=w410) -> (element=w405:dbl)
                  n223 = global read "Glob_Ref.vi" "NumDiv_rc"() -> (w404:dbl)
                  n224 = Add(x=-4.05, y=w404) -> (x+y=w402:dbl)
                  n225 = Format Into String(format string=":MEASURE:TRANGE -4.1,%#_g\n:MEASURE:CHANNEL%#_g:AVERage:VALUE?", w402, w405) -> (resulting string=w406:string)  [unwired: 2 in, 1 out]
                  n226 = call "fgv_DL950_visa.vi"("cmd"=fgv_DL950."query", "ms"=u32 110, "Initiate"=w406) -> ()  [unwired: 6 in, 3 out]
                }
                frame Enabled {
                }
              }
            }
            frame #5 {
              n227 = disable-structure shown="Disabled" {
                frame Disabled {
                  n228 = Wait (ms)(milliseconds to wait=u32 2000) -> ()  [unwired: 1 out]
                }
                frame Enabled {
                }
              }
            }
            frame #6 {
              n229 = disable-structure shown="Disabled" {
                frame Disabled {
                  n230 = call "fgv_950_parsing-arr.vi"("cmd"=rw."read") -> ("950 parsing arr 2"=w420:cluster{"950-arr 1":dbl[], "950-arr 2":dbl[]})  [unwired: 10 in]
                  n231 = Unbundle(w420) -> ("950-arr 1"=w421:dbl[], "950-arr 2"=w422:dbl[])
                  n232 = call "TrangeCalc.vi"() -> ("array"=w419:dbl[])  [unwired: 7 in, 3 out]
                  n233 = Build Array (concatenate)(w421, w422, w419) -> (w414:dbl[])
                  n234 = global write "Global 1.vi" "da950_array"(w414) -> ()
                  n235 = call "fgv_DL950_data.vi"("cmd"=rw."read") -> ("DL950 wfm 2"=w415:T26)  [unwired: 9 in, 1 out]
                  n236 = Bundle By Name(cluster=w415, "da950_array"=w414) -> (w413:T26)
                  n237 = call "fgv_DL950_data.vi"("cmd"=rw."write", "DL950 wfm"=w413) -> ()  [unwired: 8 in, 2 out]
                }
                frame Enabled {
                }
              }
            }
          }
        }
        frame "B1" {
          n238 = stacked-sequence {
            seq-local: [w425 _ _ _ _ _ _] -> [_ w433 _ _ _ _ _]
            seq-local: [_ w431 _ _ _ _ _] -> [_ _ _ w449 _ _ _]
            tunnel: w423 -> [w426 _ _ _ w458 _ _]
            frame #0 {
              n239 = Index Array(array=dbl[] [9.0, 10.0, 11.0, 12.0, 13.0, 14.0], index=w426) -> (element=w427:dbl)
              n240 = Wait (ms)(milliseconds to wait=u32 500) -> ()  [unwired: 1 out]
              n241 = Format Into String(format string=":MEASURE:CHANNEL%#_g:AVERage:VALUE?", w427) -> (resulting string=w425:string)  [unwired: 2 in, 1 out]
            }
            frame #1 {
              n242 = Concatenate Strings(":TRIGGER:POSITION?\n:TIMebase:TDIV?\n:MEASURE:CHANNEL1:RISE:VALUE?\n:MEASURE:CHANNEL2:RISE:VALUE?\n:MEASURE:CHANNEL6:FALL:VALUE?\n:MEASURE:CHANNEL5:RMS:VALUE?\n:MEASURE:CHANNEL6:RMS:VALUE?\n:MEASURE:CHANNEL5:PNUMber:VALUE?" ("String"), "\n", w433) -> (w432:string)
              n243 = Wait (ms)(milliseconds to wait=u32 200) -> ()  [unwired: 1 out]
              n244 = call "fgv_DL950_visa.vi"("cmd"=fgv_DL950."query", "ms"=u32 20, "Initiate"=w432) -> ("error out"=w436:errorcluster)  [unwired: 6 in, 2 out]
              n245 = call "TrangeCalc.vi"("error in (no error)"=w436) -> ("T2"=w445:dbl, "T1"=w444:dbl, "array"=w431:dbl[])  [unwired: 6 in, 1 out]
              n246 = Format Into String(format string=":MEASURE:TRANGE %#_g,%#_g", w444, w445) -> (resulting string=w437:string)  [unwired: 2 in, 1 out]
              n247 = call "fgv_DL950_visa.vi"("cmd"=fgv_DL950."query", "ms"=u32 20, "Initiate"=w437) -> ()  [unwired: 6 in, 3 out]
            }
            frame #2 {
              n248 = Wait (ms)(milliseconds to wait=u32 2500) -> ()  [unwired: 1 out]
            }
            frame #3 {
              n249 = call "fgv_DL950_visa.vi"("cmd"=fgv_DL950."query", "ms"=u32 200, "Initiate"=":MEASURE:CHANNEL3:AVERage:VALUE?\n:MEASURE:CHANNEL4:AVERage:VALUE?\n:MEASURE:CHANNEL6:AVERage:VALUE?" ("format string")) -> ("error out"=w455:errorcluster)  [unwired: 6 in, 2 out]
              n250 = call "TrangeCalc.vi"("error in (no error)"=w455) -> ("array"=w448:dbl[])  [unwired: 6 in, 3 out]
              n251 = Build Array (concatenate)(w449, w448) -> (w447:dbl[])
              n252 = call "fgv_DL950_data.vi"("cmd"=rw."read") -> ("DL950 wfm 2"=w451:T26)  [unwired: 9 in, 1 out]
              n253 = Bundle By Name(cluster=w451, "da950_array"=w447) -> (w450:T26)
              n254 = call "fgv_DL950_data.vi"("cmd"=rw."write", "DL950 wfm"=w450) -> ()  [unwired: 8 in, 2 out]
            }
            frame #4 {
              n255 = disable-structure shown="Disabled" {
                disable-tunnel: w458 -> [w467 _]
                frame Disabled {
                  n256 = Index Array(array=dbl[] [9.0, 10.0, 11.0, 12.0, 13.0, 14.0], index=w467) -> (element=w462:dbl)
                  n257 = global read "Glob_Ref.vi" "NumDiv_rc"() -> (w461:dbl)
                  n258 = Add(x=-4.05, y=w461) -> (x+y=w459:dbl)
                  n259 = Format Into String(format string=":MEASURE:TRANGE -4.1,%#_g\n:MEASURE:CHANNEL%#_g:AVERage:VALUE?", w459, w462) -> (resulting string=w463:string)  [unwired: 2 in, 1 out]
                  n260 = call "fgv_DL950_visa.vi"("cmd"=fgv_DL950."query", "ms"=u32 110, "Initiate"=w463) -> ()  [unwired: 6 in, 3 out]
                }
                frame Enabled {
                }
              }
            }
            frame #5 {
              n261 = disable-structure shown="Disabled" {
                frame Disabled {
                  n262 = Wait (ms)(milliseconds to wait=u32 2000) -> ()  [unwired: 1 out]
                }
                frame Enabled {
                }
              }
            }
            frame #6 {
              n263 = disable-structure shown="Disabled" {
                frame Disabled {
                  n264 = call "fgv_950_parsing-arr.vi"("cmd"=rw."read") -> ("950 parsing arr 2"=w477:cluster{"950-arr 1":dbl[], "950-arr 2":dbl[]})  [unwired: 10 in]
                  n265 = Unbundle(w477) -> ("950-arr 1"=w478:dbl[], "950-arr 2"=w479:dbl[])
                  n266 = call "TrangeCalc.vi"() -> ("array"=w476:dbl[])  [unwired: 7 in, 3 out]
                  n267 = Build Array (concatenate)(w478, w479, w476) -> (w471:dbl[])
                  n268 = global write "Global 1.vi" "da950_array"(w471) -> ()
                  n269 = call "fgv_DL950_data.vi"("cmd"=rw."read") -> ("DL950 wfm 2"=w472:T26)  [unwired: 9 in, 1 out]
                  n270 = Bundle By Name(cluster=w472, "da950_array"=w471) -> (w470:T26)
                  n271 = call "fgv_DL950_data.vi"("cmd"=rw."write", "DL950 wfm"=w470) -> ()  [unwired: 8 in, 2 out]
                }
                frame Enabled {
                }
              }
            }
          }
        }
        frame "B2" {
          n272 = call "Stall Data Flow.vim"("value in"=w482, "milliseconds to wait"=u32 2500) -> ("value out"=w481:errorcluster)  [unwired: 1 out]
          n273 = Index Array(array=dbl[] [9.0, 10.0, 11.0, 12.0, 13.0, 14.0], index=w486) -> (element=w489:dbl)
          n274 = Format Into String(format string=":MEASURE:CHANNEL5:PNUMber:VALUE?\n:MEASURE:CHANNEL6:PNUMber:VALUE?\n:MEASURE:CHANNEL4:RMS:VALUE?\n:MEASURE:CHANNEL5:RMS:VALUE?\n:MEASURE:CHANNEL6:RMS:VALUE?\n:MEASURE:CHANNEL%#_g:AVERage:VALUE?" ("String"), w489) -> (resulting string=w485:string)  [unwired: 2 in, 1 out]
          n275 = call "fgv_DL950_visa.vi"("cmd"=fgv_DL950."query", "error in"=w481, "ms"=u32 100, "Initiate"=w485) -> ("error out"=w490:errorcluster)  [unwired: 5 in, 2 out]
          n276 = call "Stall Data Flow.vim"("value in"=w490, "milliseconds to wait"=u32 100) -> ("value out"=w484:errorcluster)  [unwired: 1 out]
          n277 = call "TrangeCalc.vi"("error in (no error)"=w484) -> ("error out"=w480:errorcluster, "array"=w493:dbl[])  [unwired: 6 in, 2 out]
          n278 = call "fgv_950_parsing-arr.vi"("cmd"=rw."read") -> ("950 parsing arr 2"=w499:cluster{"950-arr 1":dbl[], "950-arr 2":dbl[]})  [unwired: 10 in]
          n279 = Bundle By Name(cluster=w499, "950-arr 1"=w493) -> (w498:cluster{"950-arr 1":dbl[], "950-arr 2":dbl[]})
          n280 = call "fgv_DL950_data.vi"("cmd"=rw."read") -> ("DL950 wfm 2"=w495:T26)  [unwired: 9 in, 1 out]
          n281 = Bundle By Name(cluster=w495, "da950_array"=w493) -> (w494:T26)
          n282 = call "fgv_950_parsing-arr.vi"("cmd"=rw."write", "950 parsing arr"=w498) -> ()  [unwired: 9 in, 1 out]
          n283 = call "fgv_DL950_data.vi"("cmd"=rw."write", "DL950 wfm"=w494) -> ()  [unwired: 8 in, 2 out]
        }
        frame "B3" {
          n284 = call "Stall Data Flow.vim"("value in"=w505, "milliseconds to wait"=u32 2500) -> ("value out"=w504:errorcluster)  [unwired: 1 out]
          n285 = Index Array(array=dbl[] [9.0, 10.0, 11.0, 12.0, 13.0, 14.0], index=w509) -> (element=w512:dbl)
          n286 = Format Into String(format string=":MEASURE:CHANNEL5:PNUMber:VALUE?\n:MEASURE:CHANNEL7:PNUMber:VALUE?\n:MEASURE:CHANNEL3:RMS:VALUE?\n:MEASURE:CHANNEL5:RMS:VALUE?\n:MEASURE:CHANNEL7:RMS:VALUE?\n:MEASURE:CHANNEL%#_g:AVERage:VALUE?" ("String"), w512) -> (resulting string=w508:string)  [unwired: 2 in, 1 out]
          n287 = call "fgv_DL950_visa.vi"("cmd"=fgv_DL950."query", "error in"=w504, "ms"=u32 100, "Initiate"=w508) -> ("error out"=w513:errorcluster)  [unwired: 5 in, 2 out]
          n288 = call "Stall Data Flow.vim"("value in"=w513, "milliseconds to wait"=u32 100) -> ("value out"=w507:errorcluster)  [unwired: 1 out]
          n289 = call "TrangeCalc.vi"("error in (no error)"=w507) -> ("error out"=w503:errorcluster, "array"=w516:dbl[])  [unwired: 6 in, 2 out]
          n290 = call "fgv_950_parsing-arr.vi"("cmd"=rw."read") -> ("950 parsing arr 2"=w522:cluster{"950-arr 1":dbl[], "950-arr 2":dbl[]})  [unwired: 10 in]
          n291 = Bundle By Name(cluster=w522, "950-arr 1"=w516) -> (w521:cluster{"950-arr 1":dbl[], "950-arr 2":dbl[]})
          n292 = call "fgv_DL950_data.vi"("cmd"=rw."read") -> ("DL950 wfm 2"=w518:T26)  [unwired: 9 in, 1 out]
          n293 = Bundle By Name(cluster=w518, "da950_array"=w516) -> (w517:T26)
          n294 = call "fgv_950_parsing-arr.vi"("cmd"=rw."write", "950 parsing arr"=w521) -> ()  [unwired: 9 in, 1 out]
          n295 = call "fgv_DL950_data.vi"("cmd"=rw."write", "DL950 wfm"=w517) -> ()  [unwired: 8 in, 2 out]
        }
      }
      n296 = call "fgv_time-check.vi"("cmd"=cmd_timecheck."scope stop", "error in (no error)"=w180) -> ("error out"=w177:errorcluster)  [unwired: 8 in, 1 out]
    }
    frame "DL950 ready" {
      n297 = flat-sequence {
        frame #0 {
          n298 = call "fgv_ctrl-ref.vi"("cmd"=rw."read") -> ("output cluster 2"=w527:T22)  [unwired: 9 in, 1 out]
          n299 = Unbundle By Name(w527) -> ("BP4610 Config"=w526:refnum<vi>)
          n300 = property class="Clust (strict)" props=["Value"](reference=w526) -> ()  [unwired: 1 in, 3 out]
        }
        frame #1 {
          n301 = call "fgv_DL950_q.vi"("cmd"=create-rw-close."write", "data"=start."init") -> ()  [unwired: 8 in, 2 out]
        }
        frame #2 {
          n302 = Wait (ms)(milliseconds to wait=u32 400) -> ()  [unwired: 1 out]
        }
        frame #3 {
          n303 = call "fgv_DL950_q.vi"("cmd"=create-rw-close."write", "data"=start."T_single") -> ()  [unwired: 8 in, 2 out]
        }
        frame #4 {
          n304 = Wait (ms)(milliseconds to wait=u32 400) -> ()  [unwired: 1 out]
        }
        frame #5 {
          n305 = Wait (ms)(milliseconds to wait=u32 1000) -> ()  [unwired: 1 out]
        }
      }
    }
    frame "DL950 trigger" {
      n306 = call "fgv_time-check.vi"("cmd"=cmd_timecheck."scope trig start") -> ("error out"=w539:errorcluster)  [unwired: 9 in, 1 out]
      n307 = call "fgv_DL950_visa.vi"("cmd"=fgv_DL950."trigger_single", "error in"=w539) -> ("error out"=w541:errorcluster)  [unwired: 7 in, 2 out]
      n308 = flat-sequence {
        tunnel: w541 -> [w543]
        tunnel: [w543] -> w537
        frame #0 {
          n309 = Wait (ms)(milliseconds to wait=u32 500) -> ()  [unwired: 1 out]
        }
      }
      n310 = call "fgv_time-check.vi"("cmd"=cmd_timecheck."scope trig stop", "error in (no error)"=w537) -> ("error out"=w536:errorcluster)  [unwired: 8 in, 1 out]
    }
    frame "Discharge check" {
      n311 = call "fgv_time-check.vi"("cmd"=cmd_timecheck."relay dischar star") -> ("error out"=w546:errorcluster)  [unwired: 9 in, 1 out]
      n312 = Tick Count (ms)() -> (millisecond timer value=w552:u32)
      n313 = while {
        tunnel: [w561] -> w551
        tunnel: w552 -> [w564]
        tunnel: [w560] -> w547
        tunnel: w546 -> [w560]
        stop <- w567 stop-if-true
        n314 = call "fgv_AI.vi"("Mode"=system-status."Read") -> ("mean-vals"=w572:dbl[])  [unwired: 8 in, 2 out]
        n315 = Tick Count (ms)() -> (millisecond timer value=w565:u32)
        n316 = Index Array(array=w572) -> (element=w570:dbl)  [unwired: 1 in]
        n317 = Subtract(x=w565, y=w564) -> (x-y=w563:u32)
        n318 = call "fgv_stop_local.vi"("cmd"=init-r-stop."read") -> ("stop"=w559:bool)  [unwired: 9 in, 1 out]
        n319 = Less?(x=w570, y=1.0) -> (x < y?=w568:bool)
        n320 = Greater?(x=w563, y=u32 10000) -> (0:w561:bool)
        n321 = Compound Arithmetic op=OR(w561, w568, w559) -> (w567:bool)
        n322 = Wait (ms)(milliseconds to wait=u32 2) -> ()  [unwired: 1 out]
      }
      n323 = case shown="True" w551 {
        tunnel: [w553 w554] -> w548
        tunnel: w547 -> [w553 w554]
        frame False {
        }
        frame True {
          n324 = call "fgv_status-display.vi"("Mode"=system-status."Update", "detail"="time out", "title"="Discharge") -> ()  [unwired: 8 in, 1 out]
          n325 = call "fgv_stop_local.vi"("cmd"=init-r-stop."stop") -> ()  [unwired: 9 in, 2 out]
        }
      }
      n326 = call "fgv_time-check.vi"("cmd"=cmd_timecheck."relay dischar stop", "error in (no error)"=w548) -> ("error out"=w545:errorcluster)  [unwired: 8 in, 1 out]
    }
    frame "Relay1".."Relay6" {
      n327 = flat-sequence {
        tunnel: w581 -> [w583]
        tunnel: [w583] -> w579
        tunnel: w577 -> [w582]
        tunnel: [w582] -> w576
        tunnel: [w597] -> w580
        tunnel: w579 -> [w597]
        tunnel: w576 -> [w596]
        tunnel: [w596] -> w575
        tunnel: w580 -> [w611]
        tunnel: [w611] -> w578
        tunnel: w575 -> [w610]
        tunnel: [w610] -> w574
        tunnel: w578 -> [w626]
        tunnel: w574 -> [w625]
        frame #0 {
          n328 = case shown="\"Relay3\"" w582 {
            tunnel: w583 -> [_ _ _ _ _ _ _ _ _ _ w584 w586 w588 w590 w592 w594 _ _ _ _]
            frame "DL950 ready", Default {
            }
            frame "DL950 clear" {
            }
            frame "DL950 trigger" {
            }
            frame "DL950 read" {
            }
            frame "AO 12v" {
            }
            frame "AO wave" {
            }
            frame "AO 0v" {
            }
            frame "relay all-off" {
            }
            frame "Discharge check" {
            }
            frame "Discharge" {
            }
            frame "Relay1" {
              n329 = call "sub ch-val-global.vi"("Relay"=cnt_Relay."R_in1", "onoff"=w584) -> ()  [unwired: 10 in]
            }
            frame "Relay2" {
              n330 = call "sub ch-val-global.vi"("Relay"=cnt_Relay."R_in2", "onoff"=w586) -> ()  [unwired: 10 in]
            }
            frame "Relay3" {
              n331 = call "sub ch-val-global.vi"("Relay"=cnt_Relay."R_in3", "onoff"=w588) -> ()  [unwired: 10 in]
            }
            frame "Relay4" {
              n332 = call "sub ch-val-global.vi"("Relay"=cnt_Relay."R_in4", "onoff"=w590) -> ()  [unwired: 10 in]
            }
            frame "Relay5" {
              n333 = call "sub ch-val-global.vi"("Relay"=cnt_Relay."R_in5", "onoff"=w592) -> ()  [unwired: 10 in]
            }
            frame "Relay6" {
              n334 = call "sub ch-val-global.vi"("Relay"=cnt_Relay."R_in6", "onoff"=w594) -> ()  [unwired: 10 in]
            }
            frame "BP4610 onoff" {
            }
            frame "BP4610 set" {
            }
            frame "DSP1500 set" {
            }
            frame "DSP1500 onoff" {
            }
          }
        }
        frame #1 {
          n335 = case shown="\"Relay3\"" w596 {
            tunnel: w597 -> [_ _ _ _ _ _ _ _ _ _ w598 w600 w602 w604 w606 w609 _ _ _ _]
            frame "DL950 ready", Default {
            }
            frame "DL950 clear" {
            }
            frame "DL950 trigger" {
            }
            frame "DL950 read" {
            }
            frame "AO 12v" {
            }
            frame "AO wave" {
            }
            frame "AO 0v" {
            }
            frame "relay all-off" {
            }
            frame "Discharge check" {
            }
            frame "Discharge" {
            }
            frame "Relay1" {
              n336 = call "fgv_UI-set.vi"("cmd"=UI."Relay in1", "onoff"=w598) -> ()  [unwired: 9 in, 1 out]
            }
            frame "Relay2" {
              n337 = call "fgv_UI-set.vi"("cmd"=UI."Relay in2", "onoff"=w600) -> ()  [unwired: 9 in, 1 out]
            }
            frame "Relay3" {
              n338 = call "fgv_UI-set.vi"("cmd"=UI."Relay in3", "onoff"=w602) -> ()  [unwired: 9 in, 1 out]
            }
            frame "Relay4" {
              n339 = call "fgv_UI-set.vi"("cmd"=UI."Relay in4", "onoff"=w604) -> ()  [unwired: 9 in, 1 out]
            }
            frame "Relay5" {
              n340 = call "fgv_UI-set.vi"("cmd"=UI."Relay in5", "onoff"=w606) -> ()  [unwired: 9 in, 1 out]
            }
            frame "Relay6" {
              n341 = call "fgv_UI-set.vi"("cmd"=UI."Relay in6", "onoff"=w609) -> ()  [unwired: 9 in, 1 out]
            }
            frame "BP4610 onoff" {
            }
            frame "BP4610 set" {
            }
            frame "DSP1500 set" {
            }
            frame "DSP1500 onoff" {
            }
          }
        }
        frame #2 {
          n342 = case shown="\"Relay3\"" w610 {
            tunnel: w611 -> [_ _ _ _ _ _ _ _ _ _ w612 w614 w616 w618 w620 w622 _ _ _ _]
            frame "DL950 ready", Default {
            }
            frame "DL950 clear" {
            }
            frame "DL950 trigger" {
            }
            frame "DL950 read" {
            }
            frame "AO 12v" {
            }
            frame "AO wave" {
            }
            frame "AO 0v" {
            }
            frame "relay all-off" {
            }
            frame "Discharge check" {
            }
            frame "Discharge" {
            }
            frame "Relay1" {
              n343 = call "sub ch-val-global.vi"("Relay"=cnt_Relay."R_out1", "onoff"=w612) -> ()  [unwired: 10 in]
            }
            frame "Relay2" {
              n344 = call "sub ch-val-global.vi"("Relay"=cnt_Relay."R_out2", "onoff"=w614) -> ()  [unwired: 10 in]
            }
            frame "Relay3" {
              n345 = call "sub ch-val-global.vi"("Relay"=cnt_Relay."R_out3", "onoff"=w616) -> ()  [unwired: 10 in]
            }
            frame "Relay4" {
              n346 = call "sub ch-val-global.vi"("Relay"=cnt_Relay."R_out4", "onoff"=w618) -> ()  [unwired: 10 in]
            }
            frame "Relay5" {
              n347 = call "sub ch-val-global.vi"("Relay"=cnt_Relay."R_out5", "onoff"=w620) -> ()  [unwired: 10 in]
            }
            frame "Relay6" {
              n348 = call "sub ch-val-global.vi"("Relay"=cnt_Relay."R_out6", "onoff"=w622) -> ()  [unwired: 10 in]
            }
            frame "BP4610 onoff" {
            }
            frame "BP4610 set" {
            }
            frame "DSP1500 set" {
            }
            frame "DSP1500 onoff" {
            }
          }
        }
        frame #3 {
          # "중요"
          n349 = case shown="True" TRUE {
            tunnel: w626 -> [_ w629]
            tunnel: w625 -> [_ w628]
            frame False {
            }
            frame True {
              n350 = case shown="\"Relay1\"" w628 {
                tunnel: w629 -> [_ _ _ _ _ _ _ _ _ _ w630 w632 w634 w636 w638 w641 _ _ _ _]
                frame "DL950 ready", Default {
                }
                frame "DL950 clear" {
                }
                frame "DL950 trigger" {
                }
                frame "DL950 read" {
                }
                frame "AO 12v" {
                }
                frame "AO wave" {
                }
                frame "AO 0v" {
                }
                frame "relay all-off" {
                }
                frame "Discharge check" {
                }
                frame "Discharge" {
                }
                frame "Relay1" {
                  n351 = call "fgv_UI-set.vi"("cmd"=UI."Relay out1", "onoff"=w630) -> ()  [unwired: 9 in, 1 out]
                }
                frame "Relay2" {
                  n352 = call "fgv_UI-set.vi"("cmd"=UI."Relay out2", "onoff"=w632) -> ()  [unwired: 9 in, 1 out]
                }
                frame "Relay3" {
                  n353 = call "fgv_UI-set.vi"("cmd"=UI."Relay out3", "onoff"=w634) -> ()  [unwired: 9 in, 1 out]
                }
                frame "Relay4" {
                  n354 = call "fgv_UI-set.vi"("cmd"=UI."Relay out4", "onoff"=w636) -> ()  [unwired: 9 in, 1 out]
                }
                frame "Relay5" {
                  n355 = call "fgv_UI-set.vi"("cmd"=UI."Relay out5", "onoff"=w638) -> ()  [unwired: 9 in, 1 out]
                }
                frame "Relay6" {
                  n356 = call "fgv_UI-set.vi"("cmd"=UI."Relay out6", "onoff"=w641) -> ()  [unwired: 9 in, 1 out]
                }
                frame "BP4610 onoff" {
                }
                frame "BP4610 set" {
                }
                frame "DSP1500 set" {
                }
                frame "DSP1500 onoff" {
                }
              }
            }
          }
          n357 = Wait (ms)(milliseconds to wait=u32 100) -> ()  [unwired: 1 out]
        }
      }
    }
    frame "DL950 clear" {
    }
    frame "DL950 Tsingle query" {
      n358 = call "fgv_rc-config.vi"("cmd"=rw."read") -> ("Testconfig out"=w646:T4)  [unwired: 9 in, 1 out]
      n359 = Unbundle By Name(w646) -> ("TrigPos[%]"=w644:dbl)
      n360 = case shown="\"ContR_LV\"" w651 {
        tunnel: w644 -> [_ _ _ w654 w665 _]
        tunnel: [_ _ _ w653 w664 _] -> w643
        tunnel: [_ _ _ w652 w663 _] -> w642
        frame "Register", Default {
          (unwired) 0.0 ("NumDiv_b1")
        }
        frame "RC" {
        }
        frame "Oper_LV" {
          (unwired) 0.0 ("NumDiv_b1")
        }
        frame "Oper_HV" {
          w656 = 10.0  # trigger position
          w655 = 50.0  # trigger percent
          n361 = global read "Glob_Ref.vi" "Control Signal_HV"() -> (w658:T23)
          n362 = global read "Glob_Ref.vi" "Oscilloscope_HV"() -> (w659:cluster{"Record Len":i32, "Time Div":u16})
          n363 = Subtract(x=w654, y=w655) -> (x-y=w661:dbl)
          n364 = Divide(x=w661, y=w656) -> (x/y=w662:dbl)
          n365 = call "Compute_Number.vi"("Oscilloscope"=w659, "Control Signal"=w658) -> ("NumDiv"=w660:dbl)  [unwired: 6 in, 3 out]
          n366 = Add(x=w662, y=-0.05) -> (x+y=w653:dbl)
          n367 = Add(x=w653, y=w660) -> (x+y=w652:dbl)
        }
        frame "ContR_LV" {
          w667 = 10.0  # trigger position
          w666 = 50.0  # trigger percent
          n368 = global read "Glob_Ref.vi" "Control Signal_LCR"() -> (w670:T23)
          n369 = global read "Glob_Ref.vi" "Oscilloscope_LCR"() -> (w669:cluster{"Record Len":i32, "Time Div":u16})
          n370 = Subtract(x=w665, y=w666) -> (x-y=w672:dbl)
          n371 = Divide(x=w672, y=w667) -> (x/y=w673:dbl)
          n372 = call "Compute_Number.vi"("Oscilloscope"=w669, "Control Signal"=w670) -> ("NumDiv"=w671:dbl)  [unwired: 6 in, 3 out]
          n373 = Add(x=w673, y=-0.05) -> (x+y=w664:dbl)
          n374 = Add(x=w664, y=w671) -> (x+y=w663:dbl)
        }
        frame "B1" {
        }
      }
      n375 = Format Into String(format string=":MEASURE:TRANGE %#_g,%#_g" ("String"), w643, w642) -> (resulting string=w648:string)  [unwired: 2 in, 1 out]
      n376 = call "fgv_DL950_visa.vi"("cmd"=fgv_DL950."query", "ms"=u32 50 ("query delay"), "Initiate"=w648) -> ()  [unwired: 6 in, 3 out]
    }
  }
  "error out" <- w7
  n377 = case shown="\"Discharge\"..\"BP4610 onoff\", \"DSP1500 onoff\"" "cmd" {
    selector: "cmd" -> [w674 w678]
    tunnel: "onoff" -> [_ w677]
    tunnel: [w675 w676] -> w14
    frame "DL950 ready", Default {
      n378 = Format Into String(w674) -> (resulting string=w675:string)  [unwired: 3 in, 1 out]
    }
    frame "Discharge".."BP4610 onoff", "DSP1500 onoff" {
      n379 = Format Into String(w678, w677) -> (resulting string=w676:string)  [unwired: 3 in, 1 out]
    }
  }
  n380 = call "sub_log_basic.vi"("desc"=w14, "Title"="hw-set") -> ()  [unwired: 9 in, 1 out]
